vi "Get_Data.vi"(10 "First Call?: T/F":bool, 11 "Init Position":T1(array[cluster]) {"Error Code" format="%b"; "ID" format="%x"}) -> (2 "Actual Positions":dbl[](array[numeric]), 3 "Reset Enable?":bool[](array[boolean]))   [LabVIEW 2015]
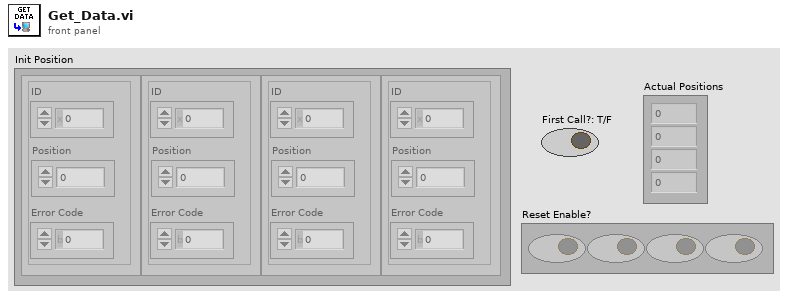
[diagram p1: front panel]
types:
  T1 = cluster{"ID":u8, "Position":u16, "Error Code":u8}[]
  T2 = cluster{"ID":u8, "Position":u16, "Error Code":u8}
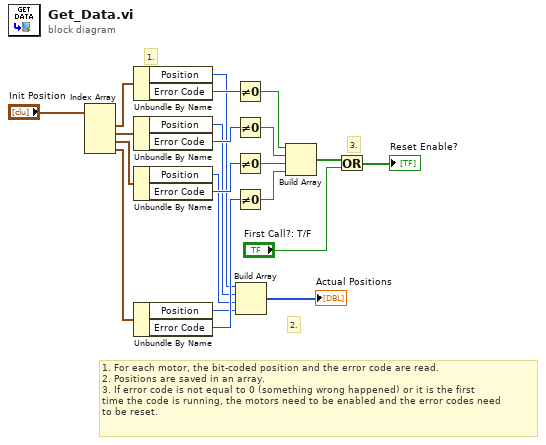
[diagram p0: block diagram]
diagram:
  # "3."
  # "2."
  # "1."
  # "1. For each motor, the bit-coded position and the error code are read.\n2. Positions are saved in an array.\n3. If error code is not equal to 0 (something wrong happened) or it is the first\ntime the code is running, the motors need to be enabled and the error codes need \nto be reset."
  n1 = Index Array(array="Init Position") -> (element #1=w2:T2, element #2=w3:T2, element #3=w4:T2, element #4=w5:T2)  [unwired: 4 in]
  n2 = Unbundle By Name(w2) -> ("Position"=w6:u16, "Error Code"=w10:u8)
  n3 = Unbundle By Name(w3) -> ("Position"=w7:u16, "Error Code"=w12:u8)
  n4 = Unbundle By Name(w4) -> ("Position"=w8:u16, "Error Code"=w14:u8)
  n5 = Unbundle By Name(w5) -> ("Position"=w9:u16, "Error Code"=w16:u8)
  n6 = Not Equal To 0?(x=w10) -> (x != 0?=w11:bool)
  n7 = Not Equal To 0?(x=w12) -> (x != 0?=w13:bool)
  n8 = Not Equal To 0?(x=w14) -> (x != 0?=w15:bool)
  n9 = Not Equal To 0?(x=w16) -> (x != 0?=w17:bool)
  n10 = Build Array(w6, w7, w8, w9) -> (→"Actual Positions":u16[])
  n11 = Build Array(w11, w13, w15, w17) -> (w18:bool[])
  n12 = Or(x=w18, y="First Call?: T/F") -> (x .or. y?=→"Reset Enable?":bool[])
